vi "SaveImages.vi"(0 "Background Image":i32[][](graph), 5 "Atoms Image":i32[][](graph), 7 "Base Filename":string, 9 "Raw Data Path":path, 11 "ImageNumber":i32) -> (4 "Background Image 2":i16[][](graph), 8 "Atoms Image 2":i16[][](graph))   [LabVIEW 2013]
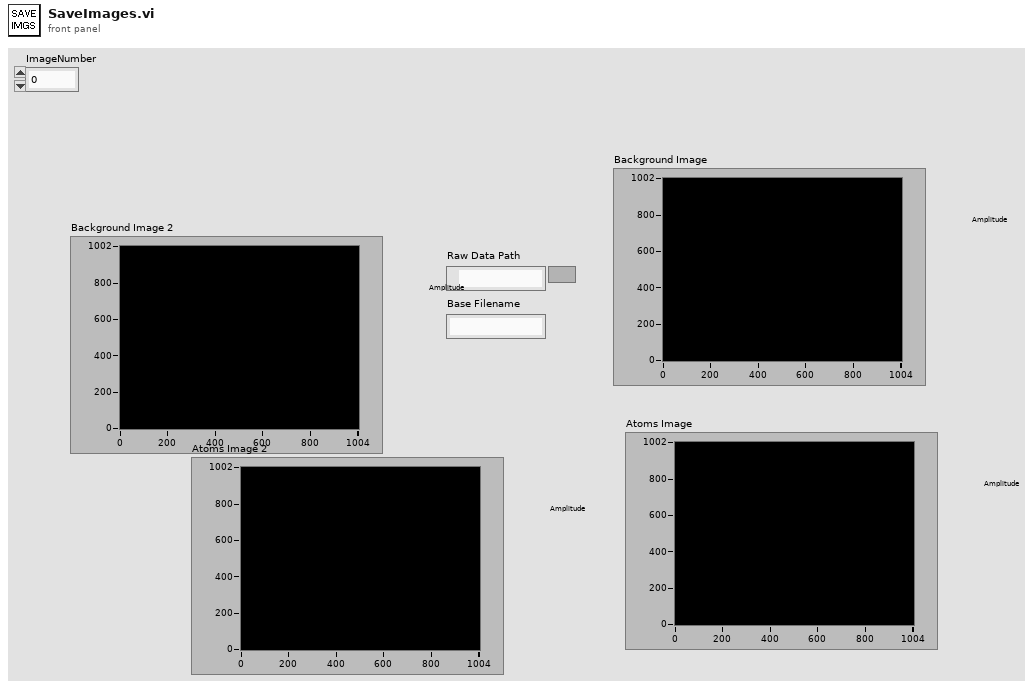
[diagram p1: front panel]
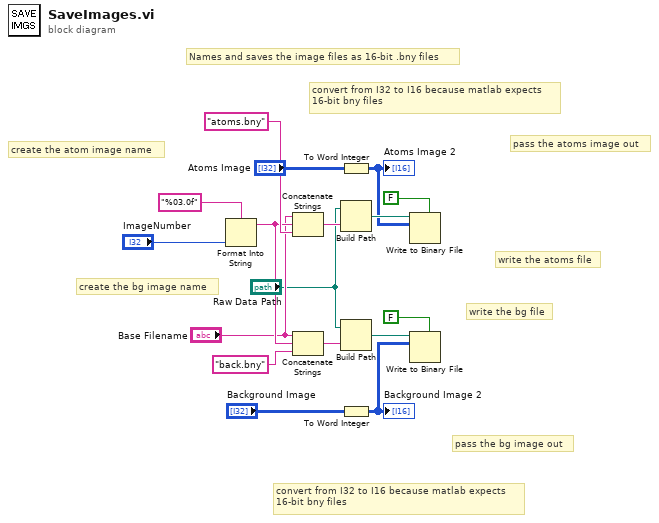
[diagram p0: block diagram]
diagram:
  # "pass the bg image out"
  # "pass the atoms image out"
  # "write the bg file"
  # "write the atoms file"
  # "convert from I32 to I16 because matlab expects\n16-bit bny files"
  # "convert from I32 to I16 because matlab expects\n16-bit bny files"
  # "create the bg image name"
  # "create the atom image name"
  # "Names and saves the image files as 16-bit .bny files"
  n1 = Format Into String(format string="%03.0f", "ImageNumber") -> (resulting string=w11:string)  [unwired: 2 in, 1 out]
  n2 = Concatenate Strings("Base Filename", w11, "atoms.bny" ("string")) -> (w9:string)
  n3 = Concatenate Strings("Base Filename", w11, "back.bny" ("string")) -> (w7:string)
  n4 = To Word Integer(number="Atoms Image") -> (16bit integer=w2:i16[][])
  "Atoms Image 2" <- w2
  n5 = Build Path(base path="Raw Data Path", name or relative path=w9) -> (appended path=w6:path)
  n6 = Build Path(base path="Raw Data Path", name or relative path=w7) -> (appended path=w5:path)
  n7 = To Word Integer(number="Background Image") -> (16bit integer=w1:i16[][])
  "Background Image 2" <- w1
  n8 = Write to Binary File(file (use dialog)=w6, data=w2, 5:FALSE ("prepend array or string size? (T)")) -> ()  [unwired: 3 in, 3 out]
  n9 = Write to Binary File(file (use dialog)=w5, data=w1, 5:FALSE ("prepend array or string size? (T)")) -> ()  [unwired: 3 in, 3 out]
